vi "Generate Error.vi"(8 "Error In":errorcluster, 10 "Arguments":string[](array[string]), 11 "DJTG Error":T1) -> (0 "Error Out":errorcluster)   [LabVIEW 2011, in "LVH-Adept.lvlib" / "DJTG.lvlib"]
uses:
  DJTG.lvlib
  Type Defs/Error.ctl
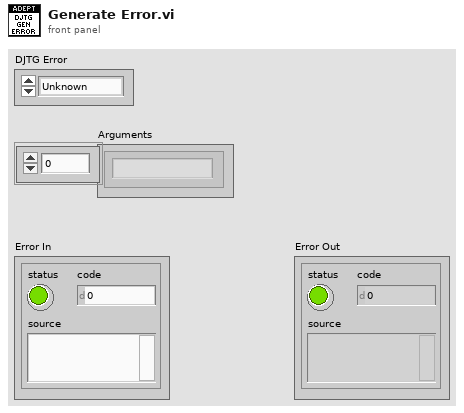
[diagram p1: front panel]
types:
  T1 = typedef "LVH-Adept.lvlib/DJTG.lvlib/Error.ctl" = enum16{"Unknown", "Enable", "PutTmsTdiBits", "GetTdoBits", "Disable", "Close", "Set Aux Reset", "Port Properties", "Get Speed", "Set Speed", "Get Port Count", "Get Batch Properties", "Enable Port", "Set Tmd Tdi Tck", "Get Tms Tdi Tdo Tck", "Put Tdi Bits", "Put Tms Bits", "Clock Tck", "Wait", "Batch", "Flash FPGA"}
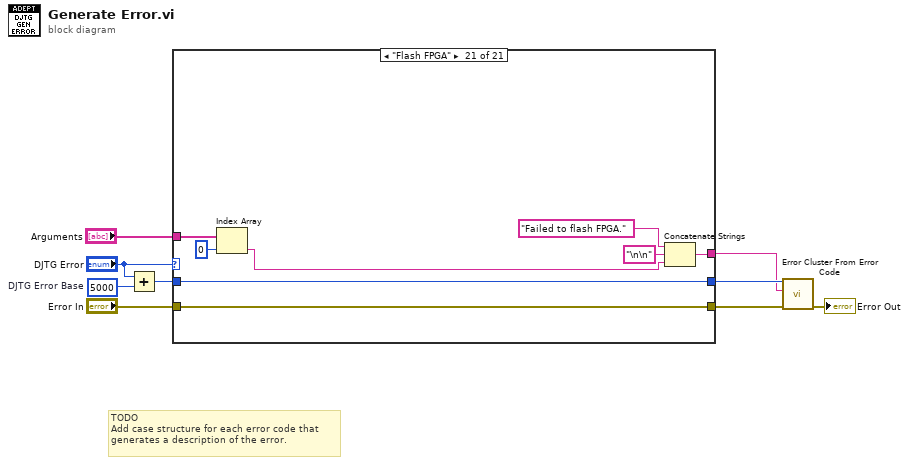
[diagram p0: block diagram]
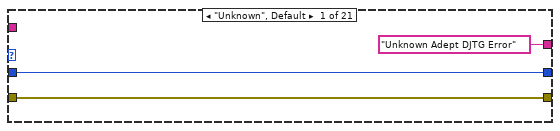
[diagram p2: hidden frame]
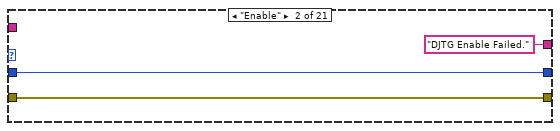
[diagram p3: hidden frame]
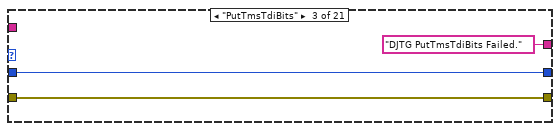
[diagram p4: hidden frame]
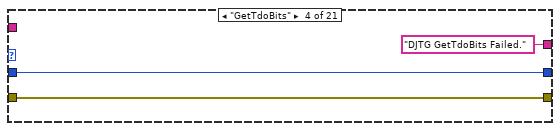
[diagram p5: hidden frame]
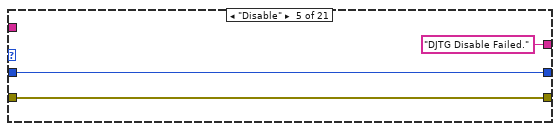
[diagram p6: hidden frame]
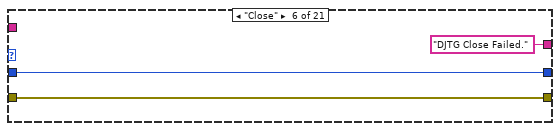
[diagram p7: hidden frame]
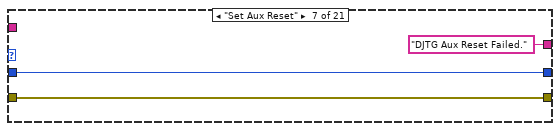
[diagram p8: hidden frame]
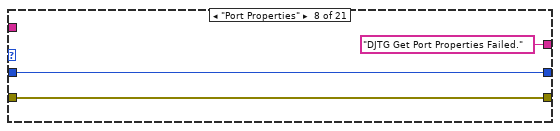
[diagram p9: hidden frame]
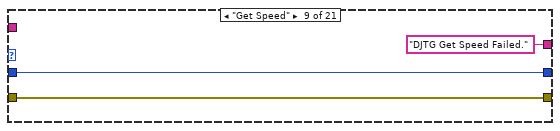
[diagram p10: hidden frame]
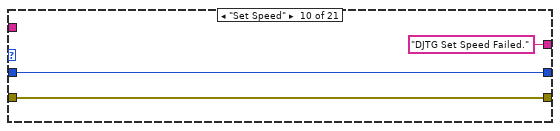
[diagram p11: hidden frame]
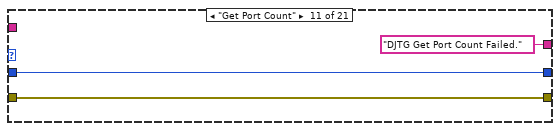
[diagram p12: hidden frame]
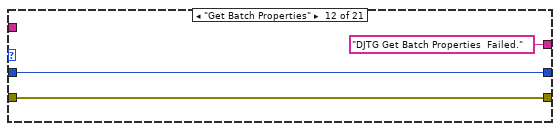
[diagram p13: hidden frame]
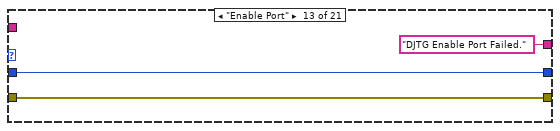
[diagram p14: hidden frame]
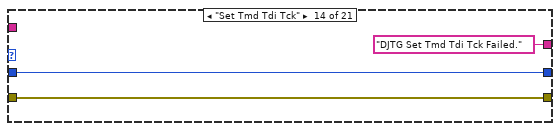
[diagram p15: hidden frame]
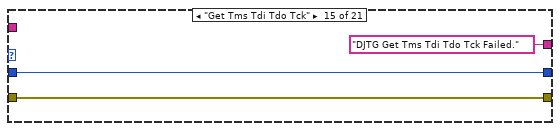
[diagram p16: hidden frame]
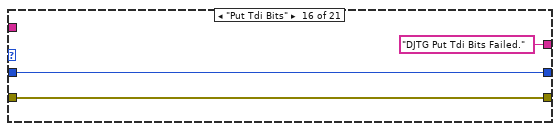
[diagram p17: hidden frame]
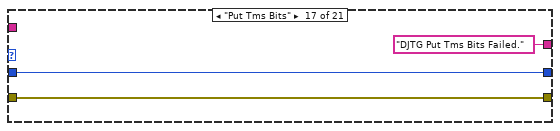
[diagram p18: hidden frame]
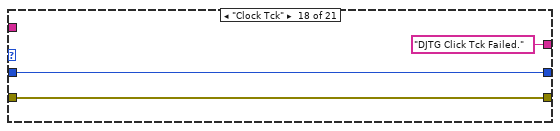
[diagram p19: hidden frame]
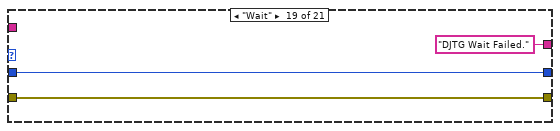
[diagram p20: hidden frame]
diagram:
  w6 = 5000  # DJTG Error Base
  # "TODO\nAdd case structure for each error code that \ngenerates a description of the error."
  n1 = Add(x="DJTG Error", y=w6) -> (x+y=w3:i32)
  n2 = case shown="\"Flash FPGA\"" "DJTG Error" {
    tunnel: [w12 w14 w17 w20 w23 w26 w29 w32 w35 w38 w41 w44 w47 w50 w53 w56 w59 w62 w65 w68 w76] -> w8
    tunnel: "Error In" -> [w12 w14 w17 w20 w23 w26 w29 w32 w35 w38 w41 w44 w47 w50 w53 w56 w59 w62 w65 w68 w76]
    tunnel: [w10 w15 w18 w21 w24 w27 w30 w33 w36 w39 w42 w45 w48 w51 w54 w57 w60 w63 w66 w69 w77] -> w5
    tunnel: ["Unknown Adept DJTG Error" "DJTG Enable Failed." "DJTG PutTmsTdiBits Failed." "DJTG GetTdoBits Failed." "DJTG Disable Failed." "DJTG Close Failed." "DJTG Aux Reset Failed." "DJTG Get Port Properties Failed." "DJTG Get Speed Failed." "DJTG Set Speed Failed." "DJTG Get Port Count Failed." "DJTG Get Batch Properties  Failed." "DJTG Enable Port Failed." "DJTG Set Tmd Tdi Tck Failed." "DJTG Get Tms Tdi Tdo Tck Failed." "DJTG Put Tdi Bits Failed." "DJTG Put Tms Bits Failed." "DJTG Click Tck Failed." "DJTG Wait Failed." "DJTG Batch Failed." w75] -> w4
    tunnel: w3 -> [w10 w15 w18 w21 w24 w27 w30 w33 w36 w39 w42 w45 w48 w51 w54 w57 w60 w63 w66 w69 w77]
    tunnel: "Arguments" -> [_ _ _ _ _ _ _ _ _ _ _ _ _ _ _ _ _ _ _ _ w74]
    frame "Unknown", Default {
    }
    frame "Enable" {
    }
    frame "PutTmsTdiBits" {
    }
    frame "GetTdoBits" {
    }
    frame "Disable" {
    }
    frame "Close" {
    }
    frame "Set Aux Reset" {
    }
    frame "Port Properties" {
    }
    frame "Get Speed" {
    }
    frame "Set Speed" {
    }
    frame "Get Port Count" {
    }
    frame "Get Batch Properties" {
    }
    frame "Enable Port" {
    }
    frame "Set Tmd Tdi Tck" {
    }
    frame "Get Tms Tdi Tdo Tck" {
    }
    frame "Put Tdi Bits" {
    }
    frame "Put Tms Bits" {
    }
    frame "Clock Tck" {
    }
    frame "Wait" {
    }
    frame "Batch" {
    }
    frame "Flash FPGA" {
      n3 = Index Array(array=w74, index=0) -> (element=w71:string)
      n4 = Concatenate Strings("Failed to flash FPGA.", "\n\n" ("string"), w71) -> (w75:string)
    }
  }
  n5 = call <vilib>:"Error Cluster From Error Code.vi"("error in (no error)"=w8, "error message (\"\")"=w4, "error code (0)"=w5) -> ("error out"=→"Error Out":errorcluster)  [unwired: 6 in]
